vi "Refresh RPC Listbox.vi"(5 "_RailP Summary Table":refnum<vi>, 7 "Mode":T1, 8 "Sync-B":T4, 9 "Sync-A":T4, 10 "PWM-B":T6={"Sensor"={"Name"="", "Unit"="", "Value"=0.0}, "Setpoint"=0.0, "PWM-A_Indicators"={"IMV"={"Current_Calc"=0.0, "DutyCyc_PIDOut"=0.7671859, "DutyCyc_MaxCalc"=0.0, "DutyCyc_Des"=0.7671859}, "HPV"={"Current_Calc"=0.0, "DutyCyc_TblOut"=0.7671859, "DutyCyc_MaxCalc"=0.0, "DutyCyc_Des"=0.7671859}}, "PWM-A_IMVChannelIndex"=0, "PWM-A_HPVChannelIndex"=0, "Fault"=FALSE, "Enable"=FALSE} {"PWM-A_IMVChannelIndex" items=["Select IMV"=-1, "IMV--HH 1"=0, "IMV--HH 2"=1, "IMV--HH 3"=2, "IMV--HH 4"=3, "IMV--HH 5"=4, "IMV--HH 6"=5, "IMV--HH 7"=6, "IMV--HH 8"=7, "IMV--HH 9"=8, "IMV--HH 10"=9, "IMV--HH 11"=10, "IMV--HH 12"=11]; "PWM-A_HPVChannelIndex" items=["Select HPV"=-1, "HPV--HH 1"=0, "HPV--HH 2"=1, "HPV--HH 3"=2, "HPV--HH 4"=3, "HPV--HH 5"=4, "HPV--HH 6"=5, "HPV--HH 7"=6, "HPV--HH 8"=7, "HPV--HH 9"=8, "HPV--HH 10"=9, "HPV--HH 11"=10, "HPV--HH 12"=11]; "PWM-A_Indicators"."HPV"."DutyCyc_Des" format="%#.3g"; "PWM-A_Indicators"."HPV"."DutyCyc_MaxCalc" max=50 format="%#.3g"; "PWM-A_Indicators"."HPV"."DutyCyc_TblOut" format="%#.3g"; "PWM-A_Indicators"."HPV"."Current_Calc" min=0 max=0.2 step=0.001 format="%#.3f"; "PWM-A_Indicators"."IMV"."DutyCyc_Des" format="%#.3g"; "PWM-A_Indicators"."IMV"."DutyCyc_MaxCalc" max=50 format="%#.3g"; "PWM-A_Indicators"."IMV"."DutyCyc_PIDOut" format="%#.3g"; "PWM-A_Indicators"."IMV"."Current_Calc" min=0 max=0.2 step=0.001 format="%#.3f"}, 11 "PWM-A":T6={"Sensor"={"Name"="", "Unit"="", "Value"=0.0}, "Setpoint"=0.0, "PWM-A_Indicators"={"IMV"={"Current_Calc"=0.0, "DutyCyc_PIDOut"=0.7671859, "DutyCyc_MaxCalc"=0.0, "DutyCyc_Des"=0.7671859}, "HPV"={"Current_Calc"=0.0, "DutyCyc_TblOut"=0.7671859, "DutyCyc_MaxCalc"=0.0, "DutyCyc_Des"=0.7671859}}, "PWM-A_IMVChannelIndex"=0, "PWM-A_HPVChannelIndex"=0, "Fault"=FALSE, "Enable"=FALSE} {"PWM-A_IMVChannelIndex" items=["Select IMV"=-1, "IMV--HH 1"=0, "IMV--HH 2"=1, "IMV--HH 3"=2, "IMV--HH 4"=3, "IMV--HH 5"=4, "IMV--HH 6"=5, "IMV--HH 7"=6, "IMV--HH 8"=7, "IMV--HH 9"=8, "IMV--HH 10"=9, "IMV--HH 11"=10, "IMV--HH 12"=11]; "PWM-A_HPVChannelIndex" items=["Select HPV"=-1, "HPV--HH 1"=0, "HPV--HH 2"=1, "HPV--HH 3"=2, "HPV--HH 4"=3, "HPV--HH 5"=4, "HPV--HH 6"=5, "HPV--HH 7"=6, "HPV--HH 8"=7, "HPV--HH 9"=8, "HPV--HH 10"=9, "HPV--HH 11"=10, "HPV--HH 12"=11]; "PWM-A_Indicators"."HPV"."DutyCyc_Des" format="%#.3g"; "PWM-A_Indicators"."HPV"."DutyCyc_MaxCalc" max=50 format="%#.3g"; "PWM-A_Indicators"."HPV"."DutyCyc_TblOut" format="%#.3g"; "PWM-A_Indicators"."HPV"."Current_Calc" min=0 max=0.2 step=0.001 format="%#.3f"; "PWM-A_Indicators"."IMV"."DutyCyc_Des" format="%#.3g"; "PWM-A_Indicators"."IMV"."DutyCyc_MaxCalc" max=50 format="%#.3g"; "PWM-A_Indicators"."IMV"."DutyCyc_PIDOut" format="%#.3g"; "PWM-A_Indicators"."IMV"."Current_Calc" min=0 max=0.2 step=0.001 format="%#.3f"}) -> ()   [LabVIEW 2016]
uses:
  Shared/Typedefs/Engine-Channel.ctl
  Shared/Typedefs/Engine-RPC-PWM-Indicators.ctl
  Shared/Typedefs/Engine-RPC-Sync-Indicators.ctl
  Shared/Typedefs/Engine-RPC-Modes.ctl
  <vilib>/Utility/miscctls.llb/LVRowAndColumnTypeDef.ctl
  Shared/DSI-Shared.lvlib
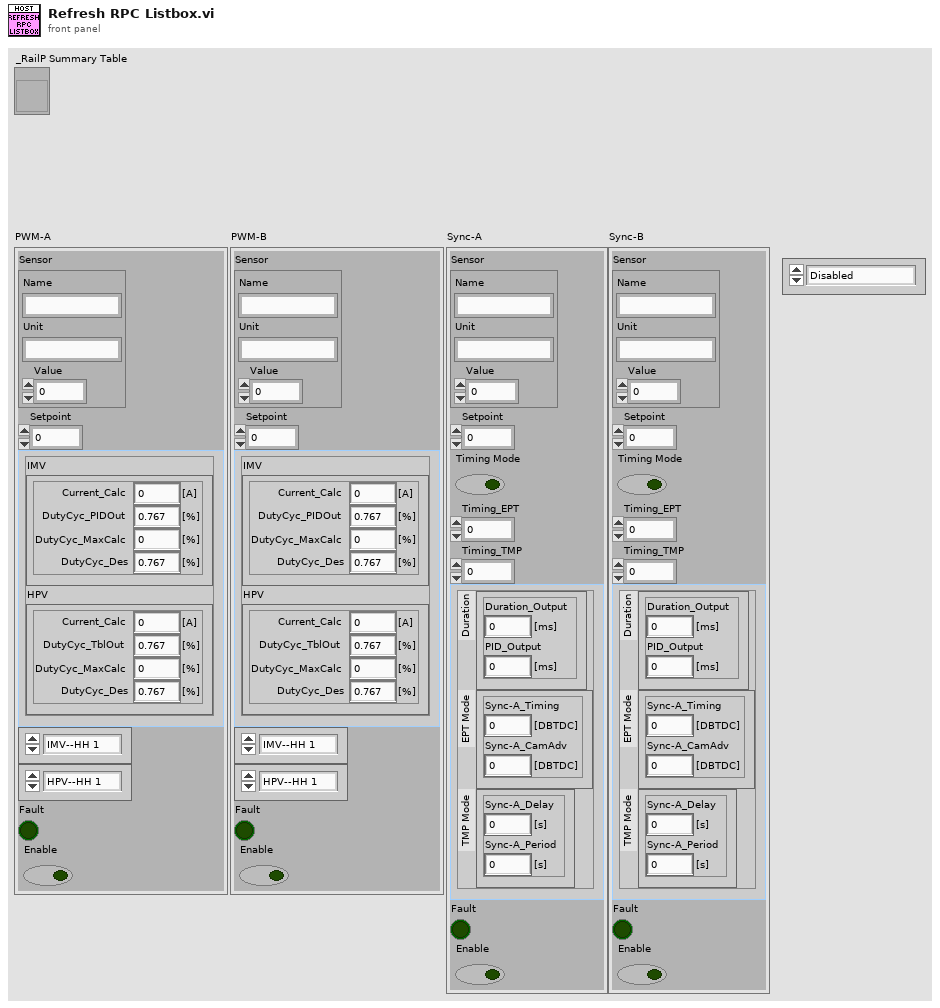
[diagram p1: front panel]
types:
  T1 = typedef "DSI-Shared.lvlib/Engine-RPC-Modes.ctl" = enum8{"Disabled", "DSI - PWM Pumps", "DSI - Sync Pumps"}
  T2 = typedef "DSI-Shared.lvlib/Engine-Channel.ctl" = cluster{"Name":string, "Unit":string, "Value":sgl}
  T3 = typedef "DSI-Shared.lvlib/Engine-RPC-Sync-Indicators.ctl" = cluster{"Duration":cluster{"Duration_Output":sgl, "PID_Output":sgl}, "EPT Mode":cluster{"Sync-A_Timing":sgl, "Sync-A_CamAdv":sgl}, "TMP Mode":cluster{"Sync-A_Delay":sgl, "Sync-A_Period":sgl}}
  T4 = cluster{"Sensor":T2, "Setpoint":sgl, "Timing Mode":bool, "Timing_EPT":sgl, "Timing_TMP":sgl, "Sync-A_Indicators":T3, "Fault":bool, "Enable":bool}
  T5 = typedef "DSI-Shared.lvlib/Engine-RPC-PWM-Indicators.ctl" = cluster{"IMV":cluster{"Current_Calc":sgl, "DutyCyc_PIDOut":sgl, "DutyCyc_MaxCalc":sgl, "DutyCyc_Des":sgl}, "HPV":cluster{"Current_Calc":sgl, "DutyCyc_TblOut":sgl, "DutyCyc_MaxCalc":sgl, "DutyCyc_Des":sgl}}
  T6 = cluster{"Sensor":T2, "Setpoint":sgl, "PWM-A_Indicators":T5, "PWM-A_IMVChannelIndex":i32, "PWM-A_HPVChannelIndex":i32, "Fault":bool, "Enable":bool}
  T7 = typedef "LVRowAndColumnTypeDef.ctl" = cluster{"Row":i32, "Column":i32}
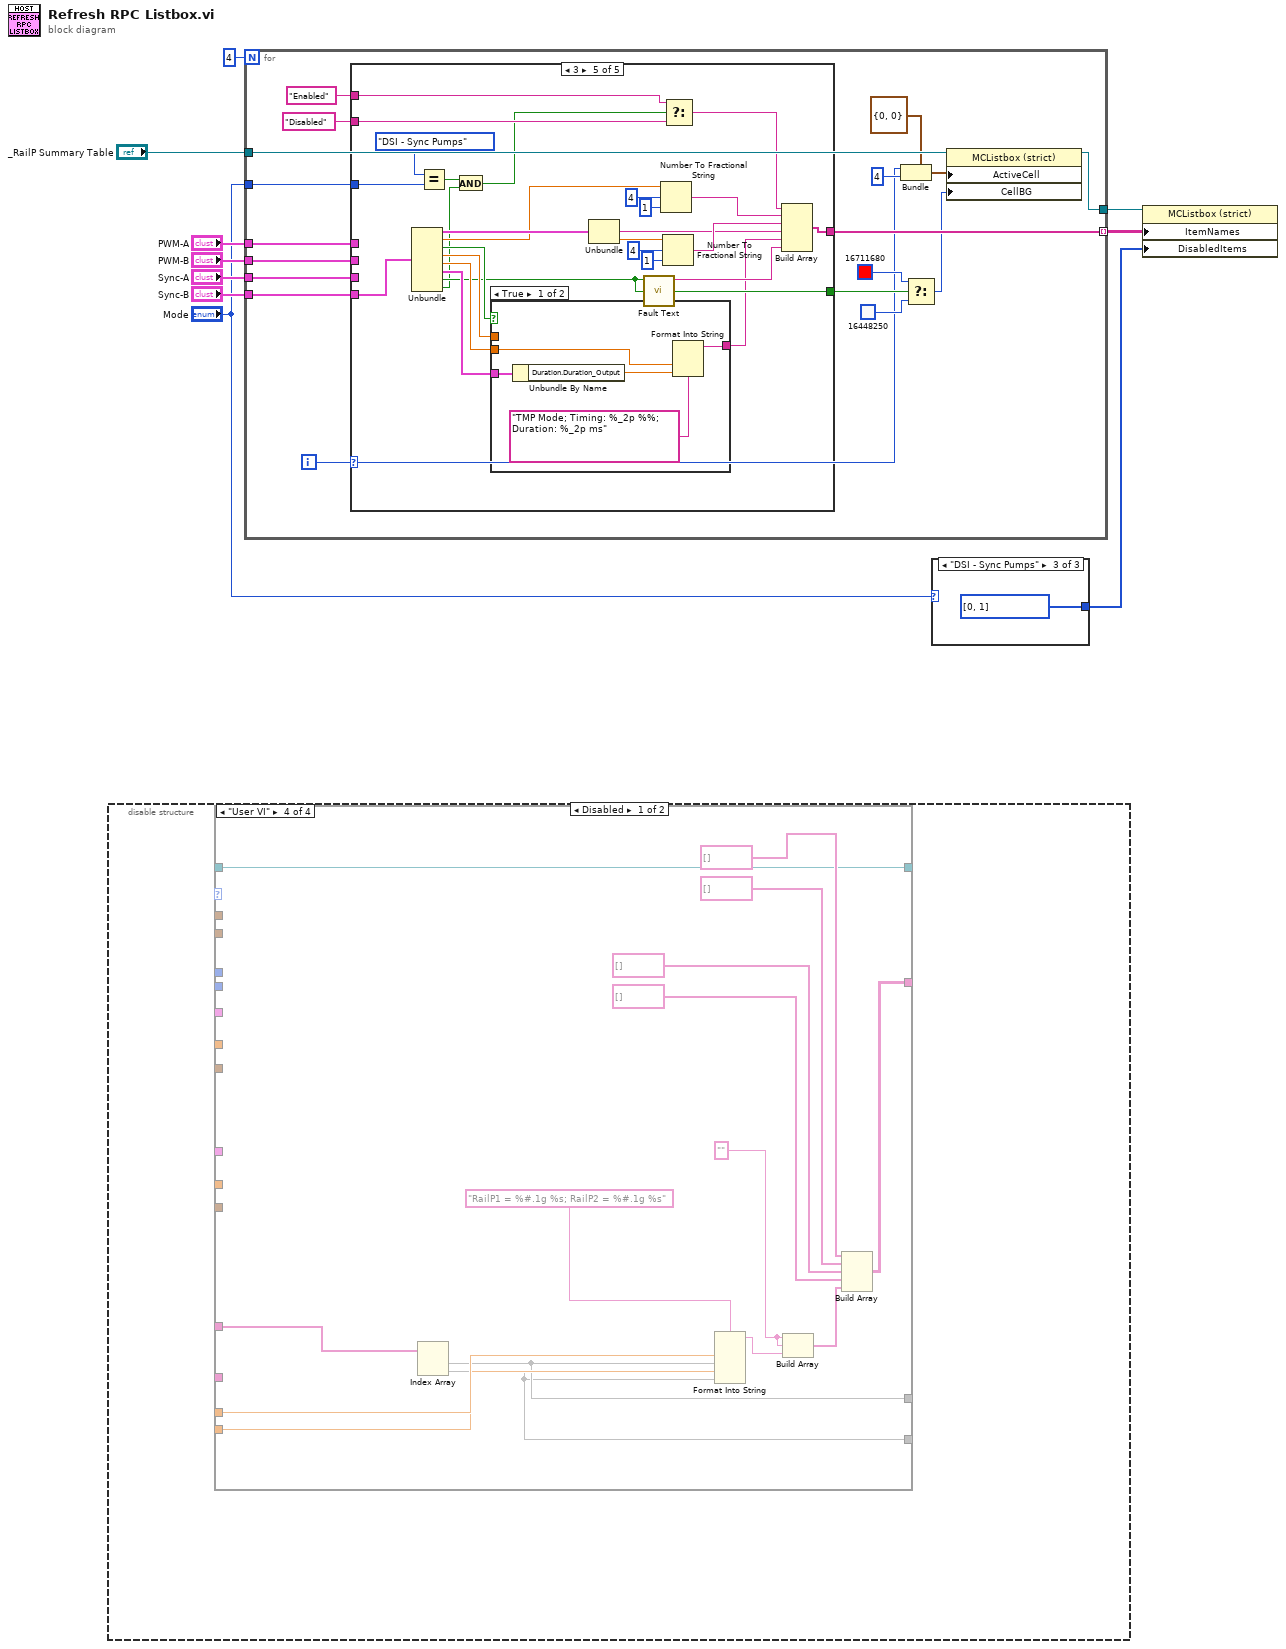
[diagram p0: block diagram]
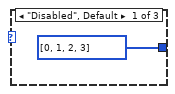
[diagram p2: hidden frame]
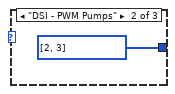
[diagram p3: hidden frame]
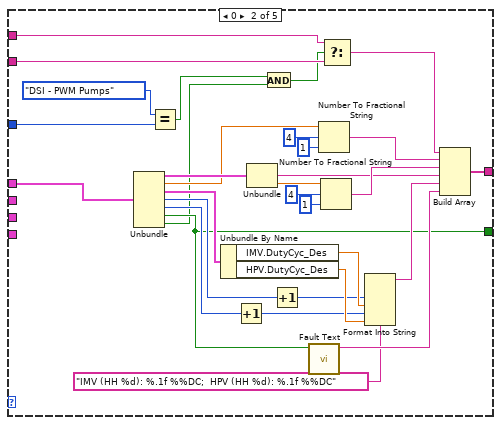
[diagram p5: hidden frame]
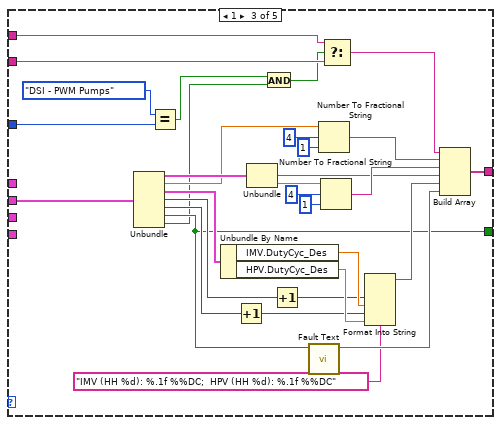
[diagram p6: hidden frame]
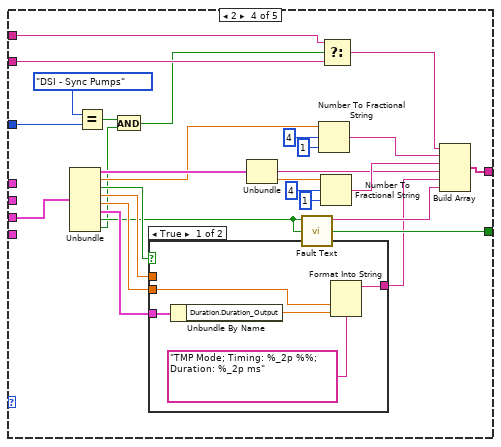
[diagram p7: hidden frame]
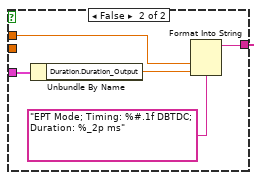
[diagram p8: hidden frame]
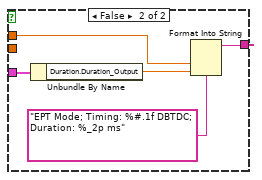
[diagram p9: hidden frame]
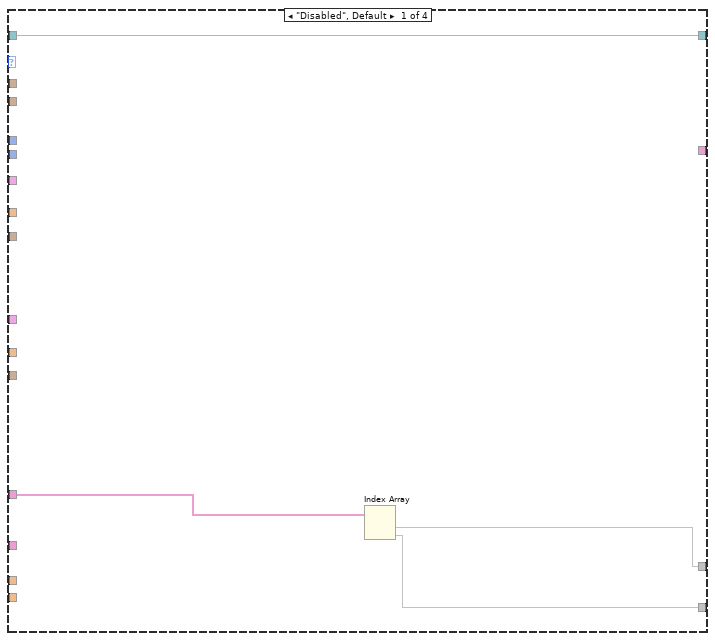
[diagram p10: hidden frame]
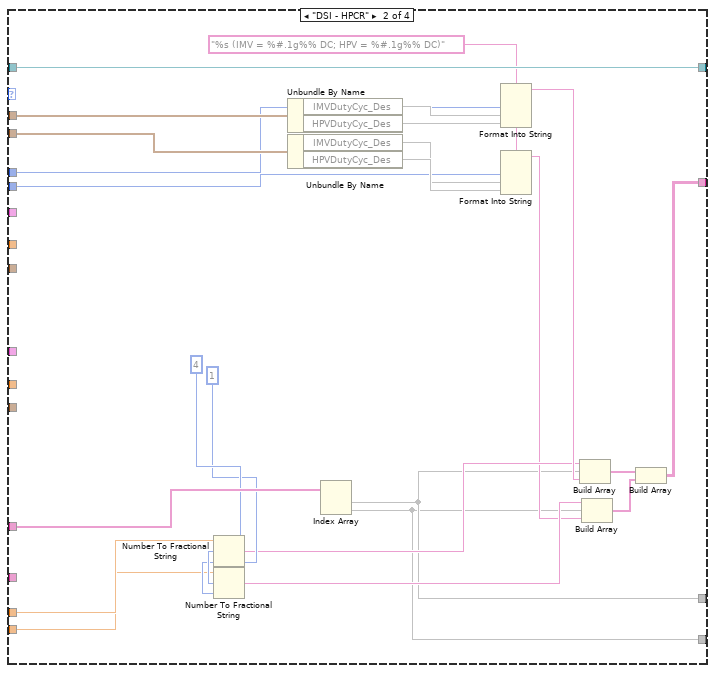
[diagram p11: hidden frame]
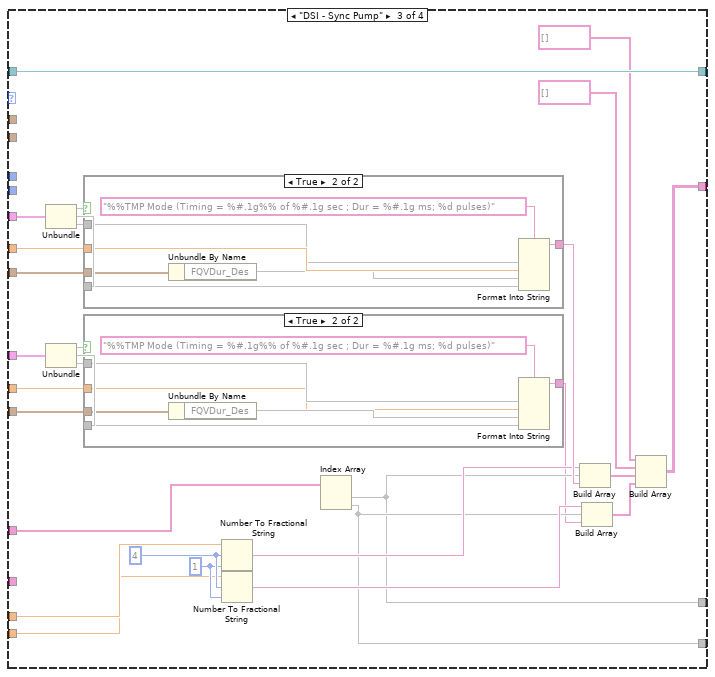
[diagram p12: hidden frame]
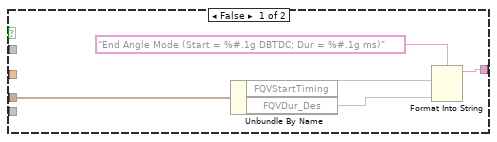
[diagram p13: hidden frame]
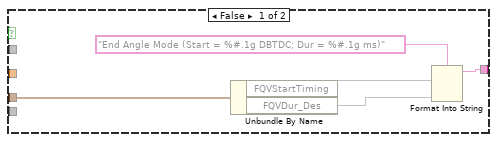
[diagram p14: hidden frame]
diagram:
  n1 = disable-structure shown="Disabled" {
    frame Disabled {
      n2 = case shown="\"User VI\"" {
        selector: _ -> [_ _ _ _]
        tunnel: _ -> [_ w36 _ _]
        tunnel: _ -> [_ w35 _ _]
        tunnel: _ -> [_ w18 _ _]
        tunnel: _ -> [_ w17 _ _]
        tunnel: _ -> [_ _ w55 _]
        tunnel: _ -> [_ _ w42 _]
        tunnel: [_ w25 w59 w105] -> _
        tunnel: _ -> [w14 w38 w67 w102]
        tunnel: [w14 w38 w67 w102] -> _
        tunnel: _ -> [w13 w37 w66 w106]
        tunnel: _ -> [_ w31 w65 w98]
        tunnel: _ -> [_ w28 w62 w97]
        tunnel: _ -> [_ _ _ _]
        tunnel: [w12 w16 w51 w93] -> _
        tunnel: [w11 w15 w52 w92] -> _
        tunnel: _ -> [_ _ w49 _]
        tunnel: _ -> [_ _ w48 _]
        tunnel: _ -> [_ _ w44 _]
        tunnel: _ -> [_ _ w40 _]
        frame "Disabled", Default {
          n3 = Index Array(array=w13) -> (element #1=w12, element #2=w11)  [unwired: 2 in]
        }
        frame "DSI - HPCR" {
          w29 = i16 1 ("precision (6)")
          w30 = i16 4 ("width (-)")
          w34 = "%s (IMV = %#.1g%% DC; HPV = %#.1g%% DC)" ("format string")
          n4 = Number To Fractional String(number=w31, width (-)=w30, precision (6)=w29) -> (F-format string=w23:string)  [unwired: 1 in]
          n5 = Number To Fractional String(number=w28, width (-)=w30, precision (6)=w29) -> (F-format string=w22:string)  [unwired: 1 in]
          n6 = Unbundle By Name(w36) -> ("IMVDutyCyc_Des"=w20, "HPVDutyCyc_Des"=w33)
          n7 = Unbundle By Name(w35) -> ("IMVDutyCyc_Des"=w19, "HPVDutyCyc_Des"=w32)
          n8 = Index Array(array=w37) -> (element #1=w16, element #2=w15)  [unwired: 2 in]
          n9 = Format Into String(format string=w34, w18, w20, w33) -> (resulting string=w24:string)  [unwired: 2 in, 1 out]
          n10 = Format Into String(format string=w34, w17, w19, w32) -> (resulting string=w21:string)  [unwired: 2 in, 1 out]
          n11 = Build Array(w23, w16, w24) -> (w27:string[])
          n12 = Build Array(w22, w15, w21) -> (w26:string[])
          n13 = Build Array(w27, w26) -> (w25:string[][])
        }
        frame "DSI - Sync Pump" {
          w63 = i16 1 ("precision (6)")
          w64 = i16 4 ("width (-)")
          n14 = Unbundle(w49) -> ("PumpA|Test%Mode"=w50, "PumpA|Pulses"=w46, "PumpA|Timingpct"=w47)
          n15 = Unbundle(w44) -> ("PumpB|Test%Mode"=w43, "PumpB|Pulses"=w39, "PumpB|Timingpct"=w41)
          n16 = case shown="True" w50 {
            tunnel: [w84 w91] -> w58
            tunnel: w55 -> [w83 w87]
            tunnel: w48 -> [_ w89]
            tunnel: w47 -> [_ w88]
            tunnel: w46 -> [_ w85]
            frame False {
              n17 = Unbundle By Name(w83) -> ("FQVStartTiming"=w82, "FQVDur_Des"=w81)
              n18 = Format Into String(format string="End Angle Mode (Start = %#.1g DBTDC; Dur = %#.1g ms)", w82, w81) -> (resulting string=w84:string)  [unwired: 2 in, 1 out]
            }
            frame True {
              n19 = Unbundle By Name(w87) -> ("FQVDur_Des"=w86)
              n20 = Format Into String(format string="%%TMP Mode (Timing = %#.1g%% of %#.1g sec ; Dur = %#.1g ms; %d pulses)", w88, w89, w86, w85) -> (resulting string=w91:string)  [unwired: 2 in, 1 out]
            }
          }
          n21 = case shown="True" w43 {
            tunnel: [w72 w79] -> w45
            tunnel: w42 -> [w71 w76]
            tunnel: w41 -> [_ w77]
            tunnel: w39 -> [_ w74]
            tunnel: w40 -> [_ w73]
            frame False {
              n22 = Unbundle By Name(w71) -> ("FQVStartTiming"=w70, "FQVDur_Des"=w69)
              n23 = Format Into String(format string="End Angle Mode (Start = %#.1g DBTDC; Dur = %#.1g ms)", w70, w69) -> (resulting string=w72:string)  [unwired: 2 in, 1 out]
            }
            frame True {
              n24 = Unbundle By Name(w76) -> ("FQVDur_Des"=w75)
              n25 = Format Into String(format string="%%TMP Mode (Timing = %#.1g%% of %#.1g sec ; Dur = %#.1g ms; %d pulses)", w77, w73, w75, w74) -> (resulting string=w79:string)  [unwired: 2 in, 1 out]
            }
          }
          n26 = Number To Fractional String(number=w65, width (-)=w64, precision (6)=w63) -> (F-format string=w57:string)  [unwired: 1 in]
          n27 = Number To Fractional String(number=w62, width (-)=w64, precision (6)=w63) -> (F-format string=w56:string)  [unwired: 1 in]
          n28 = Index Array(array=w66) -> (element #1=w51, element #2=w52)  [unwired: 2 in]
          n29 = Build Array(w57, w51, w58) -> (w61:string[])
          n30 = Build Array(w56, w52, w45) -> (w60:string[])
          n31 = Build Array(string[] [], string[] [], w61, w60) -> (w59:string[][])
        }
        frame "User VI" {
          w95 = "" ("format string")
          n32 = Index Array(array=w106) -> (element #1=w93, element #2=w92)  [unwired: 2 in]
          n33 = Format Into String(format string="RailP1 = %#.1g %s; RailP2 = %#.1g %s", w98, w93, w97, w92) -> (resulting string=w94:string)  [unwired: 2 in, 1 out]
          n34 = Build Array(w95, w95, w94) -> (w96:string[])
          n35 = Build Array(string[] [], string[] [], string[] [], string[] [], w96) -> (w105:string[][])
        }
      }
    }
    frame Enabled {
    }
  }
  n36 = for {
    N: 4 -> [_]
    tunnel: "PWM-A" -> [w124]
    tunnel: "PWM-B" -> [w123]
    tunnel: "Sync-A" -> [w122]
    tunnel: "Sync-B" -> [w121]
    tunnel: [w120] -> w6 mode=indexing
    tunnel: "_RailP Summary Table" -> [w119]
    tunnel: [w111] -> w3
    tunnel: "Mode" -> [w107]
    i -> [w110]
    n37 = case shown="3" w110 {
      tunnel: w124 -> [_ w155 _ _ _]
      tunnel: w123 -> [_ _ w156 _ _]
      tunnel: w122 -> [_ _ _ w187 _]
      tunnel: w121 -> [_ _ _ _ w229]
      tunnel: [_ w145 w177 w204 w241] -> w120
      tunnel: [_ w133 w165 w197 w234] -> w112
      tunnel: "Enabled" ("format string") -> [_ w132 w164 w194 w231]
      tunnel: "Disabled" ("format string") -> [_ w131 w163 w193 w230]
      tunnel: w107 -> [_ w128 w160 w191 w227]
      frame -1, Default {
      }
      frame 0 {
        n38 = Unbundle(w155) -> ("Sensor"=w140:T2, "Setpoint"=w139:sgl, "PWM-A_Indicators"=w138:T5, "PWM-A_IMVChannelIndex"=w137:i32, "PWM-A_HPVChannelIndex"=w136:i32, "Fault"=w133:bool, "Enable"=w126:bool)
        n39 = Equal?(x=Engine-RPC-Modes."DSI - PWM Pumps" ("Mode"), y=w128) -> (x = y?=w125:bool)
        n40 = Unbundle By Name(w138) -> ("IMV.DutyCyc_Des"=w142:sgl, "HPV.DutyCyc_Des"=w141:sgl)
        n41 = Increment(x=w136) -> (x+1=w134:i32)
        n42 = Unbundle(w140) -> ("Unit"=w147:string, "Value"=w149:sgl)  [unwired: 1 out]
        n43 = And(x=w125, y=w126) -> (x .and. y?=w127:bool)
        n44 = Increment(x=w137) -> (x+1=w135:i32)
        n45 = call "Fault Text.vi"("Boolean"=w133) -> ("Fault / No Fault"=w146:string)  [unwired: 10 in]
        n46 = Number To Fractional String(number=w139, width (-)=i16 4, precision (6)=i16 1) -> (F-format string=w152:string)  [unwired: 1 in]
        n47 = Number To Fractional String(number=w149, width (-)=i16 4, precision (6)=i16 1) -> (F-format string=w148:string)  [unwired: 1 in]
        n48 = Select(t=w132, s=w127, f=w131) -> (s? t:f=w130:string)
        n49 = Format Into String(format string="IMV (HH %d): %.1f %%DC;  HPV (HH %d): %.1f %%DC", w135, w142, w134, w141) -> (resulting string=w143:string)  [unwired: 2 in, 1 out]
        n50 = Build Array(w130, w152, w148, w147, w143, w146) -> (w145:string[])
      }
      frame 1 {
        n51 = Unbundle(w156) -> ("Sensor"=w172:T2, "Setpoint"=w171:sgl, "PWM-A_Indicators"=w170:T5, "PWM-A_IMVChannelIndex"=w169:i32, "PWM-A_HPVChannelIndex"=w168:i32, "Fault"=w165:bool, "Enable"=w158:bool)
        n52 = Equal?(x=Engine-RPC-Modes."DSI - PWM Pumps" ("Mode"), y=w160) -> (x = y?=w157:bool)
        n53 = Unbundle By Name(w170) -> ("IMV.DutyCyc_Des"=w174:sgl, "HPV.DutyCyc_Des"=w173:sgl)
        n54 = Increment(x=w168) -> (x+1=w166:i32)
        n55 = Unbundle(w172) -> ("Unit"=w179:string, "Value"=w181:sgl)  [unwired: 1 out]
        n56 = And(x=w157, y=w158) -> (x .and. y?=w159:bool)
        n57 = Increment(x=w169) -> (x+1=w167:i32)
        n58 = call "Fault Text.vi"("Boolean"=w165) -> ("Fault / No Fault"=w178:string)  [unwired: 10 in]
        n59 = Number To Fractional String(number=w171, width (-)=i16 4, precision (6)=i16 1) -> (F-format string=w184:string)  [unwired: 1 in]
        n60 = Number To Fractional String(number=w181, width (-)=i16 4, precision (6)=i16 1) -> (F-format string=w180:string)  [unwired: 1 in]
        n61 = Select(t=w164, s=w159, f=w163) -> (s? t:f=w162:string)
        n62 = Format Into String(format string="IMV (HH %d): %.1f %%DC;  HPV (HH %d): %.1f %%DC", w167, w174, w166, w173) -> (resulting string=w175:string)  [unwired: 2 in, 1 out]
        n63 = Build Array(w162, w184, w180, w179, w175, w178) -> (w177:string[])
      }
      frame 2 {
        n64 = Unbundle(w187) -> ("Sensor"=w203:T2, "Setpoint"=w202:sgl, "Timing Mode"=w201:bool, "Timing_EPT"=w200:sgl, "Timing_TMP"=w199:sgl, "Sync-A_Indicators"=w198:T3, "Fault"=w197:bool, "Enable"=w188:bool)
        n65 = Equal?(x=Engine-RPC-Modes."DSI - Sync Pumps" ("Mode"), y=w191) -> (x = y?=w189:bool)
        n66 = And(x=w189, y=w188) -> (x .and. y?=w190:bool)
        n67 = case shown="True" w201 {
          tunnel: w198 -> [w218 w223]
          tunnel: w200 -> [_ w220]
          tunnel: w199 -> [w214 _]
          tunnel: [w215 w219] -> w196
          frame True {
            n68 = Unbundle By Name(w218) -> ("Duration.Duration_Output"=w216:sgl)
            n69 = Format Into String(format string="TMP Mode; Timing: %_2p %%; Duration: %_2p ms", w214, w216) -> (resulting string=w215:string)  [unwired: 2 in, 1 out]
          }
          frame False {
            n70 = Unbundle By Name(w223) -> ("Duration.Duration_Output"=w221:sgl)
            n71 = Format Into String(format string="EPT Mode; Timing: %#.1f DBTDC; Duration: %_2p ms", w220, w221) -> (resulting string=w219:string)  [unwired: 2 in, 1 out]
          }
        }
        n72 = Unbundle(w203) -> ("Unit"=w206:string, "Value"=w208:sgl)  [unwired: 1 out]
        n73 = call "Fault Text.vi"("Boolean"=w197) -> ("Fault / No Fault"=w205:string)  [unwired: 10 in]
        n74 = Number To Fractional String(number=w202, width (-)=i16 4, precision (6)=i16 1) -> (F-format string=w211:string)  [unwired: 1 in]
        n75 = Number To Fractional String(number=w208, width (-)=i16 4, precision (6)=i16 1) -> (F-format string=w207:string)  [unwired: 1 in]
        n76 = Select(t=w194, s=w190, f=w193) -> (s? t:f=w195:string)
        n77 = Build Array(w195, w211, w207, w206, w196, w205) -> (w204:string[])
      }
      frame 3 {
        n78 = Unbundle(w229) -> ("Sensor"=w240:T2, "Setpoint"=w239:sgl, "Timing Mode"=w238:bool, "Timing_EPT"=w237:sgl, "Timing_TMP"=w236:sgl, "Sync-A_Indicators"=w235:T3, "Fault"=w234:bool, "Enable"=w224:bool)
        n79 = Equal?(x=Engine-RPC-Modes."DSI - Sync Pumps" ("Mode"), y=w227) -> (x = y?=w225:bool)
        n80 = And(x=w225, y=w224) -> (x .and. y?=w226:bool)
        n81 = case shown="True" w238 {
          tunnel: w235 -> [w255 w260]
          tunnel: w237 -> [_ w257]
          tunnel: w236 -> [w251 _]
          tunnel: [w252 w256] -> w233
          frame True {
            n82 = Unbundle By Name(w255) -> ("Duration.Duration_Output"=w253:sgl)
            n83 = Format Into String(format string="TMP Mode; Timing: %_2p %%; Duration: %_2p ms", w251, w253) -> (resulting string=w252:string)  [unwired: 2 in, 1 out]
          }
          frame False {
            n84 = Unbundle By Name(w260) -> ("Duration.Duration_Output"=w258:sgl)
            n85 = Format Into String(format string="EPT Mode; Timing: %#.1f DBTDC; Duration: %_2p ms", w257, w258) -> (resulting string=w256:string)  [unwired: 2 in, 1 out]
          }
        }
        n86 = Unbundle(w240) -> ("Unit"=w243:string, "Value"=w245:sgl)  [unwired: 1 out]
        n87 = call "Fault Text.vi"("Boolean"=w234) -> ("Fault / No Fault"=w242:string)  [unwired: 10 in]
        n88 = Number To Fractional String(number=w239, width (-)=i16 4, precision (6)=i16 1) -> (F-format string=w248:string)  [unwired: 1 in]
        n89 = Number To Fractional String(number=w245, width (-)=i16 4, precision (6)=i16 1) -> (F-format string=w244:string)  [unwired: 1 in]
        n90 = Select(t=w231, s=w226, f=w230) -> (s? t:f=w232:string)
        n91 = Build Array(w232, w248, w244, w243, w233, w242) -> (w241:string[])
      }
    }
    n92 = Bundle(cluster=T7 {"Row"=0, "Column"=0} ("Active Cell:Active Cell"), "Row"=w110, "Column"=4) -> (w117:T7)
    n93 = Select(t=u32 16711680, s=w112, f=u32 16448250) -> (s? t:f=w113:u32)
    n94 = property class="MCListbox (strict)"(reference=w119, "ActiveCell"=w117, "CellBG"=w113) -> (reference out=w111:refnum<vi>)  [unwired: 1 in, 1 out]
  }
  n95 = case shown="\"DSI - Sync Pumps\"" "Mode" {
    tunnel: [i32[] [0, 1, 2, 3] ("Disabled Items") i32[] [2, 3] ("Disabled Items") i32[] [0, 1] ("Disabled Items")] -> w2
    frame "Disabled", Default {
    }
    frame "DSI - PWM Pumps" {
    }
    frame "DSI - Sync Pumps" {
    }
  }
  n96 = property class="MCListbox (strict)"(reference=w3, "ItemNames"=w6, "DisabledItems"=w2) -> ()  [unwired: 1 in, 2 out]
